vi "niDTS GNSS RF Test Fetch Results.vi"(0 "Template Tx Test Handle in":T2, 11 "error in (no error)":errorcluster) -> (4 "Template Tx Test Handle out":T2, 8 "Results":T1, 15 "error out":errorcluster)   [LabVIEW 2014, in "niDTS GNSS.lvlib"]
uses:
  niDTS GNSS.lvlib
  Includes/niDTS GNSS RF Test INC Handle.ctl
  Objects/BASE_class/niDTS GNSS RF Test.lvclass
  Includes/niDTS GNSS RF Test INC Results.ctl
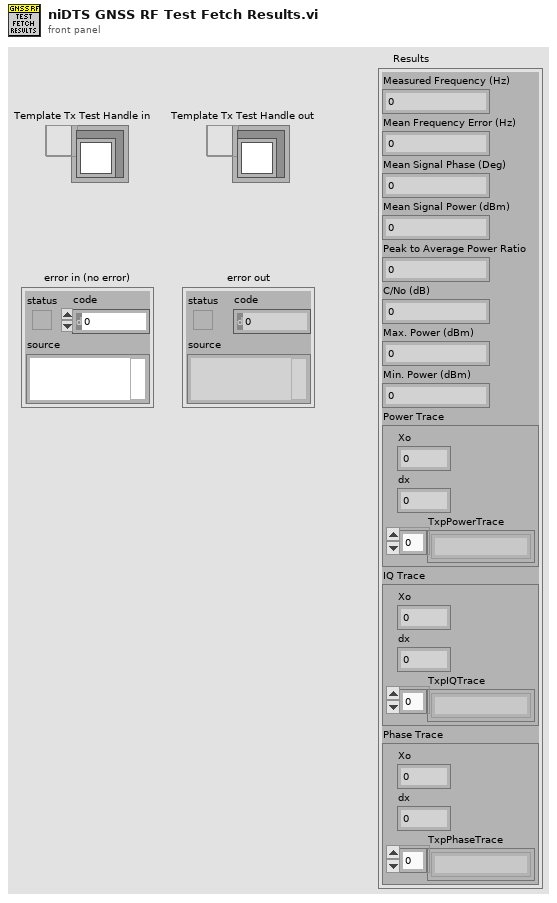
[diagram p1: front panel]
types:
  T1 = typedef "niDTS GNSS.lvlib/niDTS GNSS RF Test INC Results.ctl" = cluster{"Measured Frequency (Hz)":dbl, "Mean Frequency Error (Hz)":dbl, "Mean Signal Phase (Deg)":dbl, "Mean Signal Power (dBm)":dbl, "Peak to Average Power Ratio":dbl, "C/No (dB)":dbl, "Max. Power (dBm)":dbl, "Min. Power (dBm)":dbl, "Power Trace":cluster{"Xo":dbl, "dx":dbl, "TxpPowerTrace":string[]}, "IQ Trace":cluster{"Xo":dbl, "dx":dbl, "TxpIQTrace":string[]}, "Phase Trace":cluster{"Xo":dbl, "dx":dbl, "TxpPhaseTrace":string[]}}
  T2 = typedef "niDTS GNSS.lvlib/niDTS GNSS RF Test INC Handle.ctl" = refnum<data-value>
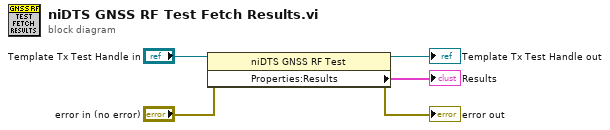
[diagram p0: block diagram]
diagram:
  n1 = property class="niDTS GNSS RF Test"(reference="Template Tx Test Handle in", error in="error in (no error)") -> (reference out=→"Template Tx Test Handle out":T2, error out=→"error out":errorcluster, "Properties:Results"=→"Results":T1)
